vi "Write Update Data MSG.vi"(8 "error in (no error)":errorcluster, 10 "DAQ Device.lvlib:Update Data MSG":refnum<class "Generic Update Data Message.lvclass">, 11 "Instr Actor in":refnum<class "Instr Actor.lvclass">) -> (0 "error out":errorcluster, 3 "Instr Actor out":refnum<class "Instr Actor.lvclass">)   [LabVIEW 2014, in "Instrument Library.lvlib" / "Instr Actor.lvclass"]
uses:
  Instr Actor.lvclass
  reusable/DAQ Device/Device/Generic Data Update Data MSG/Generic Update Data Message.lvclass
  Instr Actor.lvclass/Instr Actor.ctl
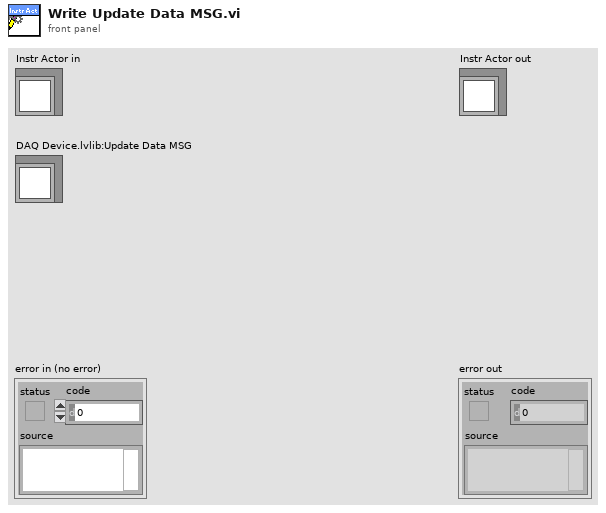
[diagram p1: front panel]
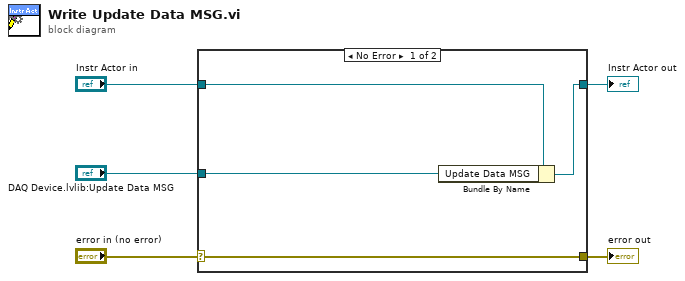
[diagram p0: block diagram]
diagram:
  n1 = case shown="No Error" "error in (no error)" {
    selector: "error in (no error)" -> [w9 w10]
    tunnel: [w9 w10] -> w4
    tunnel: [w7 w11] -> w2
    tunnel: "Instr Actor in" -> [w8 w11]
    tunnel: "DAQ Device.lvlib:Update Data MSG" -> [w6 _]
    frame No Error {
      n2 = Bundle By Name(cluster=w8, "Update Data MSG"=w6) -> (w7:refnum<class "Instr Actor.lvclass">)
    }
    frame Error {
    }
  }
  "error out" <- w4
  "Instr Actor out" <- w2
